vi "GFITS_toFits.vi"(3 "nodeID":string, 4 "ms timeout (-1)":i32=-1, 5 "response Q":string, 6 "key":string, 7 "error in (no error)":errorcluster, 8 "data":u16[](array[numeric]), 9 "eleRead":u32[](array[numeric]), 10 "location":u64, 11 "command":string) -> (0 "error out":errorcluster, 1 "response":errorcluster)   [LabVIEW 2016]
uses:
  private/vis/GFITS_imageDataStruct.ctl
panel:
  in  "cmd struct":T1
  in  "image data":T2
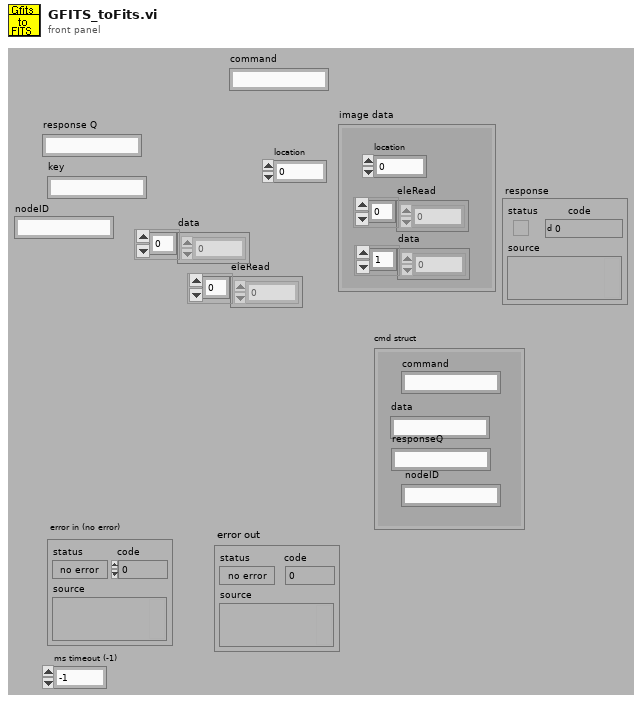
[diagram p1: front panel]
types:
  T1 = cluster{"command":string, "data":string, "responseQ":string, " nodeID":string}
  T2 = typedef "GFITS_imageDataStruct.ctl" = cluster{"location":u64, "eleRead":u32[], "data":u16[]}
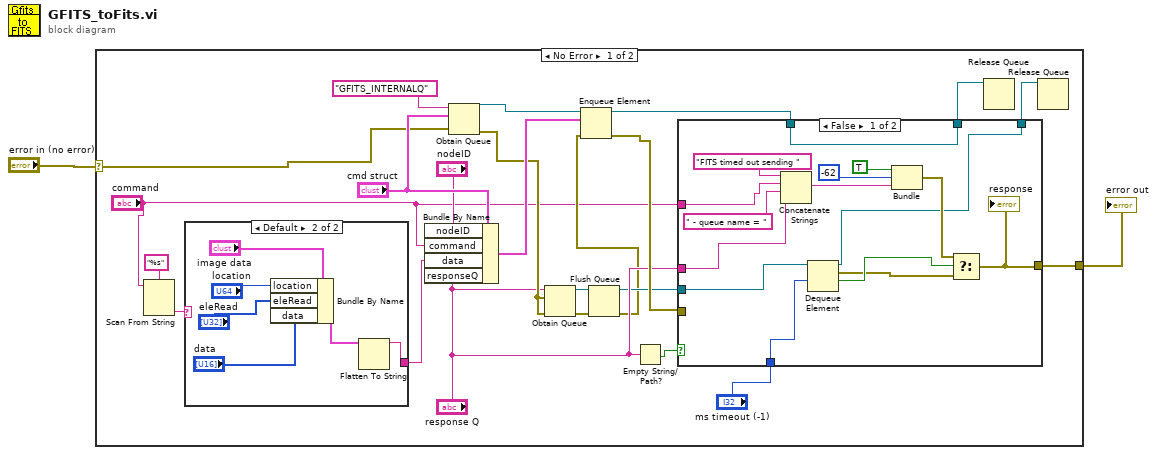
[diagram p0: block diagram]
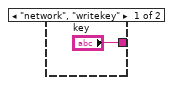
[diagram p3: hidden frame]
diagram:
  n1 = case shown="No Error" "error in (no error)" {
    selector: "error in (no error)" -> [w17 w51]
    tunnel: [w22 w51] -> w1
    frame No Error {
      n2 = Scan From String(format string="%s", input string="command") -> (output 1=w3:string)  [unwired: 2 in, 4 out]
      n3 = case shown="Default" w3 {
        tunnel: ["key" w45] -> w25
        frame "network", "writekey" {
        }
        frame Default {
          n4 = Bundle By Name(cluster="image data", "location"="location", "eleRead"="eleRead", "data"="data") -> (w46:T2)
          n5 = Flatten To String(anything=w46) -> (data string=w45:string)  [unwired: 1 in, 4 out]
        }
      }
      n6 = Bundle By Name(cluster="cmd struct", "nodeID"="nodeID", "command"="command", "data"=w25, "responseQ"="response Q") -> (w18:T1)
      n7 = Obtain Queue(name (unnamed)="GFITS_INTERNALQ", element data type="cmd struct", error in (no error)=w17) -> (queue out=w19:refnum<queue>, error out=w13:errorcluster)  [unwired: 2 in, 1 out]
      n8 = Obtain Queue(name (unnamed)="response Q", element data type=w13, error in (no error)=w13) -> (queue out=w10:refnum<queue>, error out=w9:errorcluster)  [unwired: 2 in, 1 out]
      n9 = Flush Queue(queue=w10, error in (no error)=w9) -> (queue out=w8:refnum<queue>, error out=w7:errorcluster)  [unwired: 1 out]
      n10 = Enqueue Element(queue=w19, element=w18, error in (no error)=w7) -> (queue out=w15:refnum<queue>, error out=w14:errorcluster)  [unwired: 2 out]
      n11 = Empty String/Path?(string/path="response Q") -> (empty?=w24:bool)
      n12 = case shown="False" w24 {
        tunnel: "response Q" -> [w32 _]
        tunnel: "ms timeout (-1)" -> [w29 _]
        tunnel: w14 -> [_ w43]
        tunnel: [w40 w43] -> w22
        tunnel: "command" -> [w39 _]
        tunnel: [w28 w42] -> w16
        tunnel: w15 -> [w28 w42]
        tunnel: w8 -> [w27 w41]
        tunnel: [w26 w41] -> w12
        frame False {
          n13 = Concatenate Strings("FITS timed out sending " ("source"), w39, " - queue name = ", w32) -> (w36:string)
          n14 = Dequeue Element(queue=w27, timeout in ms (-1)=w29) -> (queue out=w26:refnum<queue>, element=w30:errorcluster, timed out?=w31:bool)  [unwired: 1 in, 1 out]
          n15 = Bundle(TRUE, -62, w36) -> (w37:errorcluster)  [unwired: 1 out]
          n16 = Select(t=w37, s=w31, f=w30) -> (s? t:f=w40:errorcluster)
          "response" <- w40
        }
        frame True {
        }
      }
      n17 = Release Queue(queue=w16) -> ()  [unwired: 1 in, 4 out]
      n18 = Release Queue(queue=w12) -> ()  [unwired: 1 in, 4 out]
    }
    frame Error {
    }
  }
  "error out" <- w1
